vi "Semver.vi"(4 "Meta-Data":string[](array[string]), 6 "Pre-Release":string[](array[string]), 8 "error in (no error)":errorcluster, 9 "Patch":i32, 10 "Minor":i32, 11 "Major":i32) -> (0 "error out":errorcluster, 3 "Semver out":refnum<class "Semver.lvclass">)   [LabVIEW 2017, in "Semver.lvlib" / "Semver.lvclass"]
uses:
  Semver.lvclass
  Semver.lvclass/Semver.ctl
  <vilib>/Utility/error.llb/Error Cluster From Error Code.vi
  <vilib>/ErrorRing/Error Ring.xnode
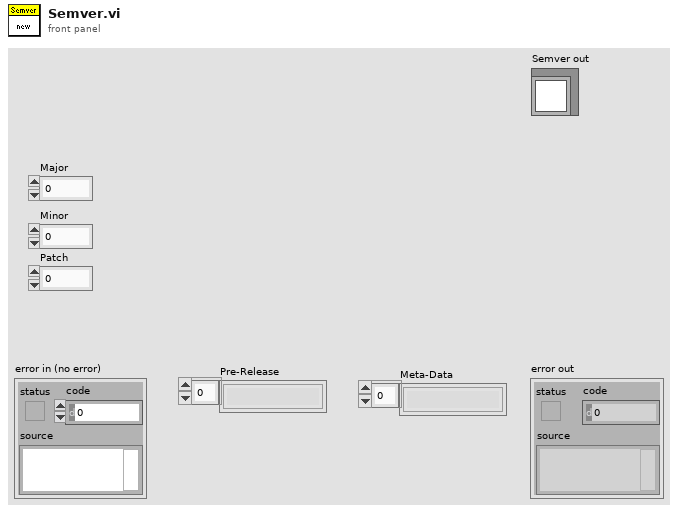
[diagram p1: front panel]
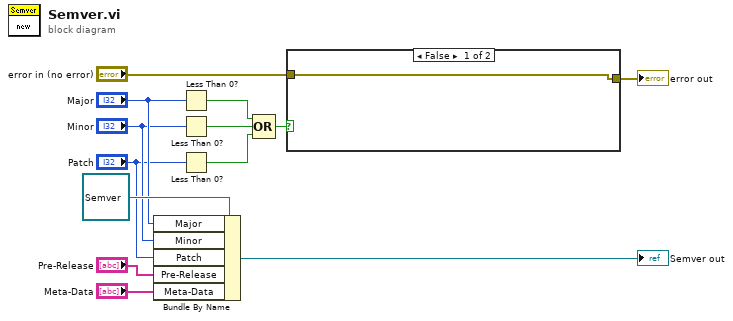
[diagram p0: block diagram]
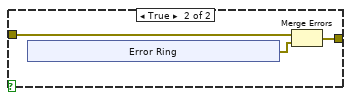
[diagram p2: hidden frame]
diagram:
  n1 = Bundle By Name(cluster=refnum<class "Semver.lvclass"> refnum ("Semver in"), "Major"="Major", "Minor"="Minor", "Patch"="Patch", "Pre-Release"="Pre-Release", "Meta-Data"="Meta-Data") -> (→"Semver out":refnum<class "Semver.lvclass">)
  n2 = Less Than 0?(x="Major") -> (x < 0?=w5:bool)
  n3 = Less Than 0?(x="Minor") -> (x < 0?=w4:bool)
  n4 = Less Than 0?(x="Patch") -> (x < 0?=w3:bool)
  n5 = Compound Arithmetic op=OR(w5, w4, w3) -> (w1:bool)
  n6 = case shown="False" w1 {
    tunnel: "error in (no error)" -> [w14 w17]
    tunnel: [w14 w16] -> w2
    frame False {
    }
    frame True {
      n7 = xnode "Error Ring"() -> ("error out"=w15:errorcluster)
      n8 = Merge Errors(w17, w15) -> (w16:errorcluster)
    }
  }
  "error out" <- w2
